vi "Measure.vi"(8 "error in (no error)":errorcluster caption="错误输入（无错误）", 11 "34461A 输入":refnum<class "34461A.lvclass">) -> (0 "error out":errorcluster caption="错误输出", 2 "Measurement":dbl, 3 "34461A 输出":refnum<class "34461A.lvclass">)   [LabVIEW 2020, in "34461A.lvlib" / "34461A.lvclass"]
uses:
  34461A.lvclass
  <instrlib>/Agilent 3446X Series/Public/Data/Read (Single Point).vi
  <instrlib>/Agilent 3446X Series/Agilent 3446X Series.lvlib
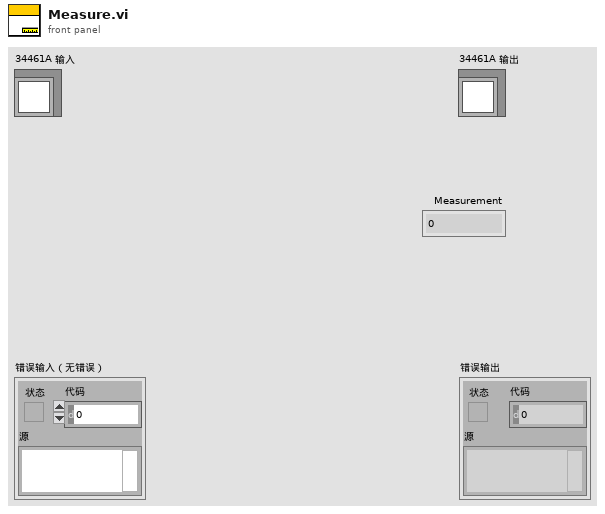
[diagram p1: front panel]
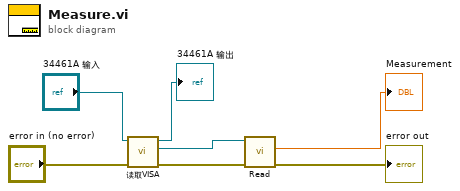
[diagram p0: block diagram]
diagram:
  n1 = call "读取VISA.vi"("error in (no error)"="error in (no error)", "数字多用表接口输入"="34461A 输入") -> ("error out"=w4:errorcluster, "VISA"=w3:refnum<visa-resource-name>, "数字多用表接口输出"=→"34461A 输出":refnum<class "34461A.lvclass">)  [unwired: 7 in]
  n2 = call-poly <instrlib>:"Read.vi"("error in (no error)"=w4, "VISA resource name"=w3) -> ("error out"=→"error out":errorcluster, "Measurement"=→"Measurement":dbl)  [unwired: 7 in, 1 out]
